vi "grabber image display panel.vi"() -> ()   [LabVIEW 2010]
panel:
  in  "overlay rectangles":T1
  in  "spilt ff/fb":bool
  in  "display volume queue":refnum<queue>
  out "XZ view":T2(plugin-control)
  out "ZY view":T2(plugin-control)
  out "XY view":T2(plugin-control)
  out "deltaZ":dbl
  out "pixel sums":cluster{"ch0 sum":u32, "ch1 sum":u32}
  in  "display channels":cluster{"CH0":bool, "CH1":bool}={"CH0"=TRUE, "CH1"=TRUE}
  out "max values from im":T3
  in  "max values":T4={"xy max"={"r max"=-1.0, "g max"=-1.0, "b max"=-1.0}, "xz max"={"r max"=-1.0, "g max"=-1.0, "b max"=-1.0}, "zy max"={"r max"=-1.0, "g max"=-1.0, "b max"=-1.0}}
  in  "turn on displays":bool=TRUE
  in  "xyz order":bool
  in  "stop":bool
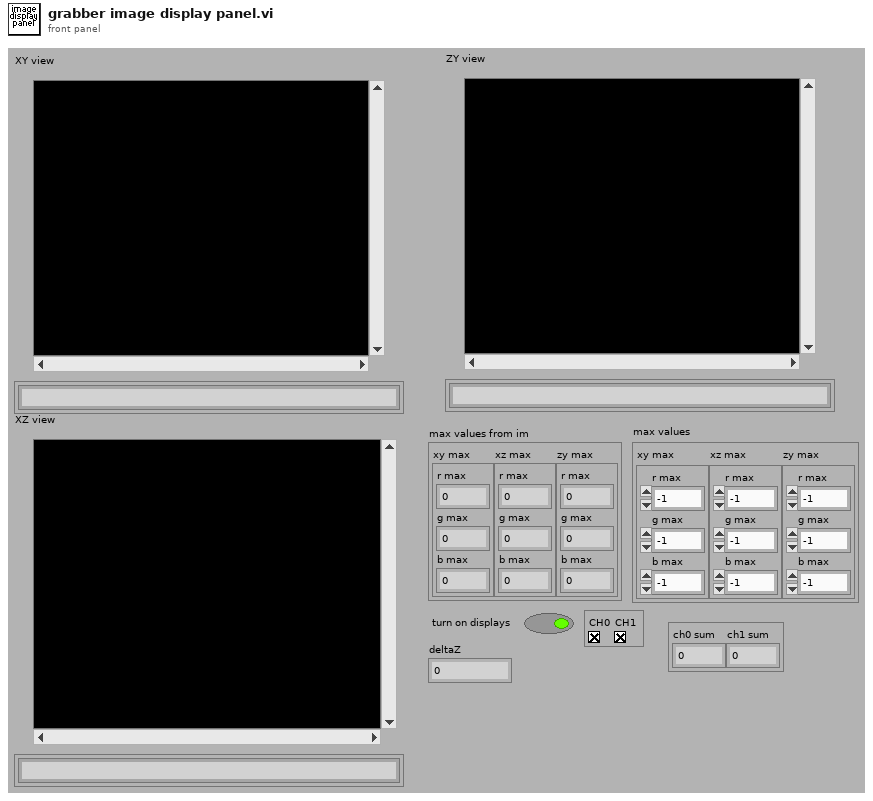
[diagram p1: front panel]
types:
  T1 = cluster{"xy box":cluster{"Left":i32, "Top":i32, "Right":i32, "Bottom":i32}, "xz box":cluster{"Left":i32, "Top":i32, "Right":i32, "Bottom":i32}, "zy box":cluster{"Left":i32, "Top":i32, "Right":i32, "Bottom":i32}}
  T2 = typedef "IMAQ Image.ctl" = refnum<image>
  T3 = cluster{"xy max":cluster{"r max":u32, "g max":u32, "b max":u32}, "xz max":cluster{"r max":u32, "g max":u32, "b max":u32}, "zy max":cluster{"r max":u32, "g max":u32, "b max":u32}}
  T4 = cluster{"xy max":cluster{"r max":dbl, "g max":dbl, "b max":dbl}, "xz max":cluster{"r max":dbl, "g max":dbl, "b max":dbl}, "zy max":cluster{"r max":dbl, "g max":dbl, "b max":dbl}}
  T5 = typedef "Image Type" = u32
  T6 = cluster{"New Image":T2, "New Image":T2, "New Image":T2}
  T7 = cluster{"ch0 volume":u32[][][], "ch1 volume":u32[][][], "ff 0+1":u32[][][], "fb 0+1":u32[][][]}
  T8 = cluster{"Image Dst Out":T2, "Image Dst Out":T2, "Image Dst Out":T2}
  T9 = cluster{"Left":i32, "Top":i32, "Right":i32, "Bottom":i32}
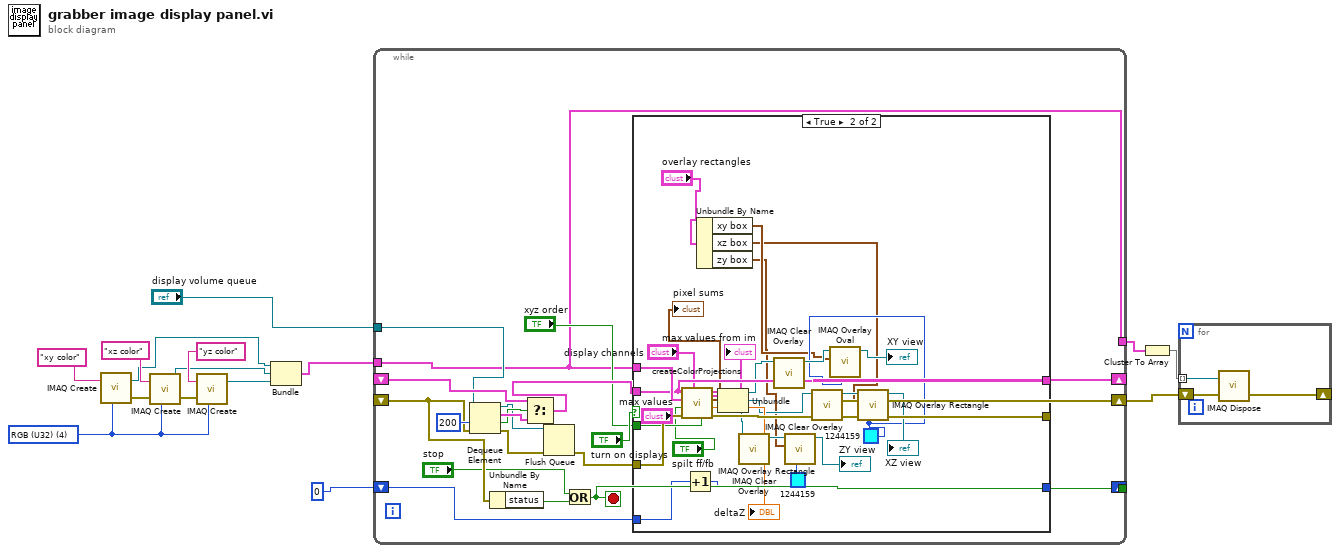
[diagram p0: block diagram]
diagram:
  w6 = T5 4 items=["Grayscale (U8)", "Grayscale (I16)", "Grayscale (SGL)", "Complex (CSG)", "RGB (U32)", "HSL (U32)", "RGB (U64)", "Grayscale (U16)"] ("Image Type")
  n1 = call "IMAQ Create"("Image Name"="xy color", "Image Type"=w6) -> ("New Image"=w9:T2, "error out"=w11:errorcluster)  [unwired: 3 in]
  n2 = call "IMAQ Create"("Image Name"="xz color", "Image Type"=w6, "error in (no error)"=w11) -> ("New Image"=w8:T2, "error out"=w10:errorcluster)  [unwired: 2 in]
  n3 = call "IMAQ Create"("Image Name"="yz color", "Image Type"=w6, "error in (no error)"=w10) -> ("New Image"=w7:T2)  [unwired: 2 in, 1 out]
  n4 = Bundle("New Image"=w9, "New Image"=w8, "New Image"=w7) -> (w5:T6)  [unwired: 1 in]
  n5 = while {
    tunnel: w5 -> [w16]
    shift-right: [w35] -> w1
    shift-left: _ -> [w31]
    tunnel: [w33] -> _
    shift-right: [w29] -> _
    shift-left: 0 -> [w30]
    shift-right: [w28] -> _
    shift-left: _ -> [w23]
    tunnel: "display volume queue" -> [w19]
    tunnel: [w16] -> w3
    stop <- w33 stop-if-true
    n6 = Dequeue Element(queue=w19, timeout in ms (-1)=200, error in (no error)=w31) -> (queue out=w20:refnum<queue>, element=w27:T7, timed out?=w26:bool, error out=w22:errorcluster)
    n7 = Unbundle By Name(w31) -> ("status"=w34:bool)
    n8 = Select(t=w23, s=w26, f=w27) -> (s? t:f=w24:T7)
    n9 = Flush Queue(queue=w20, error in (no error)=w22) -> (error out=w21:errorcluster)  [unwired: 2 out]
    n10 = Or(x="stop", y=w34) -> (x .or. y?=w33:bool)
    n11 = case shown="True" "turn on displays" {
      tunnel: w16 -> [_ w67]
      tunnel: [w38 w66] -> w35
      tunnel: w24 -> [w36 w60]
      tunnel: w21 -> [w38 w63]
      tunnel: w30 -> [w37 w62]
      tunnel: [w37 w61] -> w29
      tunnel: [w36 w60] -> w28
      tunnel: "xyz order" -> [_ w59]
      frame False {
      }
      frame True {
        w44 = u32 1244159 ("Color")
        n12 = call "createColorProjections.vi"("xyz order"=w59, "max values"="max values", "display channels"="display channels", "error in (no error)"=w63, "spilt ff/fb"="spilt ff/fb", "color ims"=w67, "volumes for display"=w60) -> ("error out"=w66:errorcluster, "deltaZ"=→"deltaZ":dbl, "pixel sums"=→"pixel sums":cluster{"ch0 sum":u32, "ch1 sum":u32}, "color ims out"=w65:T8, "max values from im"=→"max values from im":T3)
        n13 = Increment(x=w62) -> (x+1=w61:i32)
        n14 = Unbundle By Name("overlay rectangles") -> ("xy box"=w41:T9, "xz box"=w40:T9, "zy box"=w39:T9)
        n15 = Unbundle(w65) -> ("Image Dst Out"=w47:T2, "Image Dst Out"=w50:T2, "Image Dst Out"=w64:T2)
        n16 = call "IMAQ Clear Overlay"("Image"=w64) -> ("Image Out"=w53:T2)  [unwired: 9 in, 1 out]
        n17 = call "IMAQ Clear Overlay"("Image"=w47) -> ("Image Out"=w46:T2)  [unwired: 9 in, 1 out]
        n18 = call "IMAQ Overlay Rectangle"("Color"=u32 1244159, "Rectangle"=w39, "Image"=w53) -> ("Image Out"=→"ZY view":T2)  [unwired: 7 in, 1 out]
        n19 = call "IMAQ Clear Overlay"("Image"=w50) -> ("Image Out"=w49:T2)  [unwired: 9 in, 1 out]
        n20 = call "IMAQ Overlay Oval"("Color"=w44, "Bounding Rectangle"=w41, "Image"=w46) -> ("Image Out"=→"XY view":T2)  [unwired: 7 in, 1 out]
        n21 = call "IMAQ Overlay Rectangle"("Color"=w44, "Rectangle"=w40, "Image"=w49) -> ("Image Out"=→"XZ view":T2)  [unwired: 7 in, 1 out]
      }
    }
  }
  n22 = Cluster To Array(cluster=w3) -> (array=w2:T2[])
  n23 = for {
    tunnel: w2 -> [w70] mode=indexing
    shift-right: [w68] -> _
    shift-left: w1 -> [w69]
    n24 = call "IMAQ Dispose"("Image"=w70, "error in (no error)"=w69) -> ("error out"=w68:errorcluster)  [unwired: 4 in]
  }
